vi "FrameworkTestSuite_Init.vi"(8 "error in (no error)":errorcluster, 11 "reference in":refnum<class "MixedTest TestSuite.lvclass">) -> (0 "error out":errorcluster, 3 "reference out":refnum<class "MixedTest TestSuite.lvclass">)   [LabVIEW 2013, in "MixedTest TestSuite.lvclass"]
uses:
  MixedTest TestSuite.lvclass
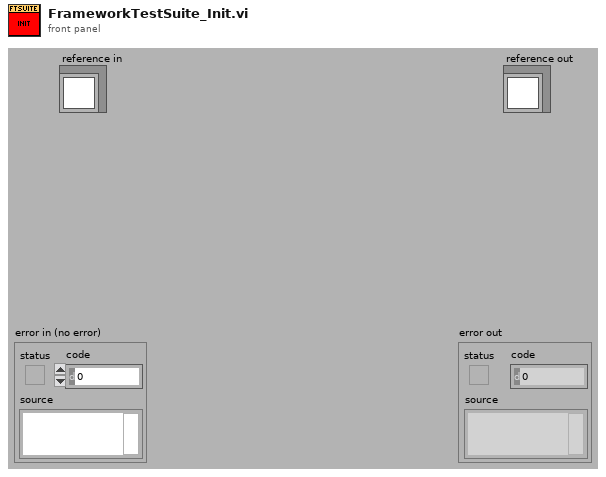
[diagram p1: front panel]
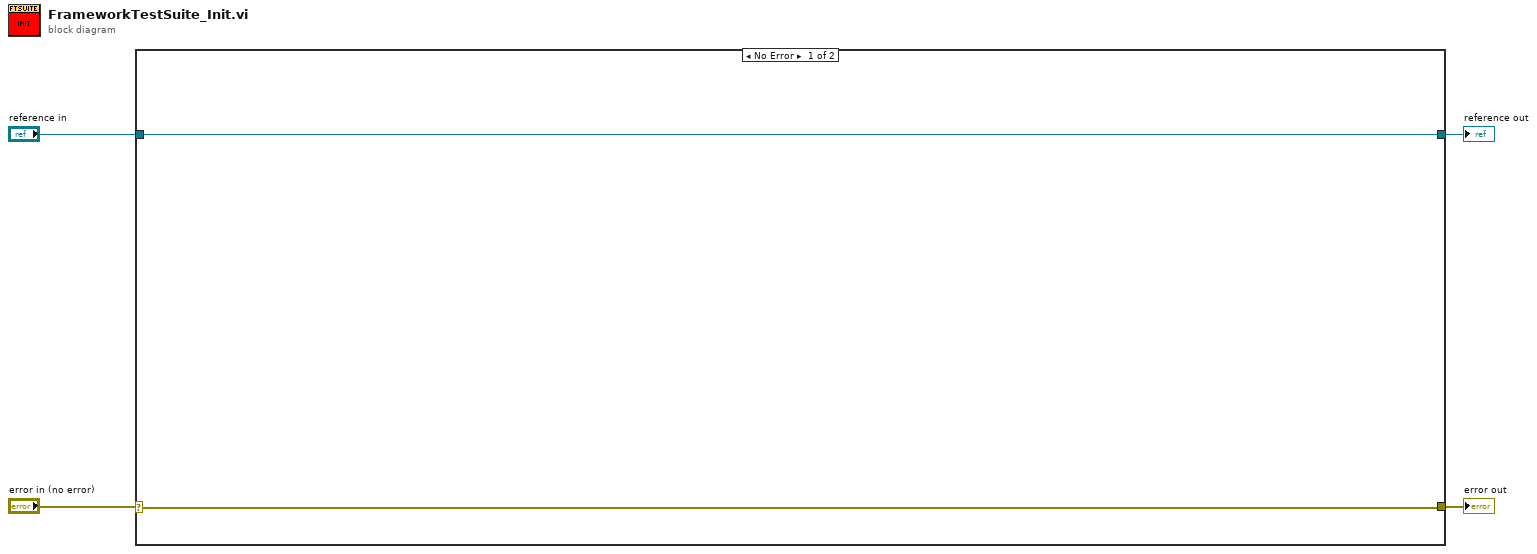
[diagram p0: block diagram]
diagram:
  n1 = case shown="No Error" "error in (no error)" {
    selector: "error in (no error)" -> [w6 w7]
    tunnel: [w5 w8] -> w4
    tunnel: "reference in" -> [w5 w8]
    tunnel: [w6 w7] -> w1
    frame No Error {
    }
    frame Error {
    }
  }
  "reference out" <- w4
  "error out" <- w1
